vi "TestOutputToFileAPI.vi"() -> ()   [LabVIEW 2014, in "OutputToFileModule.lvlib"]
uses:
  OutputToFileModule.lvlib
  EventPlugins/EventPluginBaseClass/TypeDefs/clEvtReportArray.ctl
  EventPlugins/EventPluginBaseClass/TypeDefs/clEvtReport.ctl
  NetworkImpairmentModule/PublicAPI/Arguments/Broadcasts/dblNetworkTime.ctl
  NetworkImpairmentModule/PublicAPI/Arguments/Broadcasts/dblPktLoss.ctl
  OutputToFilePlugins/OutputToFileBasePlugin/Typedefs/PmuCfgOpt.ctl
  <userlib>/NIST/ModuleAdminLib/ModuleAdmin/ModuleAdmin.lvclass
  PublicAPI/Arguments/Broadcasts/clDidInit.ctl
  <userlib>/NIST/ModuleAdminLib/ModuleAdmin/ModuleAdmin.lvclass/ModuleAdmin.ctl
  PublicAPI/Arguments/Requests/clStopArgument.ctl
  PublicAPI/Arguments/Broadcasts/clStatUpdate.ctl
  PublicAPI/Arguments/Broadcasts/clErrorRpt.ctl
  <userlib>/NIST/ModuleAdminLib/ModuleAdmin/Accessors/Read CloneRegRef.vi
  <userlib>/NIST/ModuleAdminLib/CloneRegistration/CloneRegistration.lvclass
  OutputToFilePlugins/OutputToFileBasePlugin/OutputToFileBasePlugin.lvclass
  EventPlugins/EventPluginBaseClass/EventPluginBaseClass.lvclass
  NetworkImpairmentModule/NetworkImpairmentModule.lvlib
panel:
  in  "Show Panel":bool=TRUE
  in  "btnOutputErrorFile":bool
  in  "btnReadOutputPath":bool
  out "OutputPath":path
  in  "OutputPath":path
  in  "btnWriteOutputPath":bool
  in  "btnReadPmuConfig":bool
  out "clConfigOptions":T1={"TIME_BASE"=1000000, "STN"="Bus_1", "IDCODE"=0, "rdoPolRect"=enum."Rectangular", "rdoFloatInt"=enum."Float", "PHUNIT"=1000000, "rdoFreqDfreq"=enum."Float", "CHNAM"=[], "chkCfg2Prefix"=TRUE} caption="PMU Configuration Options" {"PHUNIT" max=16777216 step=1 format="%08d"; "IDCODE" format="%02x"; "TIME_BASE" max=16777216 step=1 format="%08d"}
  in  "btnWritePmuConfig":bool
  in  "clConfigOptions 2":T1={"TIME_BASE"=1000000, "STN"="Bus_1", "IDCODE"=0, "rdoPolRect"=enum."Rectangular", "rdoFloatInt"=enum."Float", "PHUNIT"=1000000, "rdoFreqDfreq"=enum."Float", "CHNAM"=["VA"], "chkCfg2Prefix"=TRUE} caption="PMU Configuration Options" {"PHUNIT" max=16777216 step=1 format="%08d"; "IDCODE" format="%02x"; "TIME_BASE" max=16777216 step=1 format="%08d"}
  in  "btnWritePktLoss":bool
  in  "btnWriteNetTime":bool
  in  "dblPktLoss":T2
  in  "dblNetworkTime":T3
  in  "btnWriteImpairRpt":bool
  in  "clPmuImpairRptArray":T4=[{"Timestamp"=1.0, "Synx"=[99.0+0.0i], "Freq"=59.0, "ROCOF"=0.0, "ID"=0}] {"Synx" format="%#_4g"}
  in  "btnWriteEvtRpt":bool
  in  "clEvtReportArray":T4=[{"Timestamp"=1.0, "Synx"=[100.0+0.0i], "Freq"=60.0, "ROCOF"=0.0, "ID"=0}] {"Synx" format="%#_4g"}
  in  "btnReadPlugin":bool
  out "PathToPluginIniFile":path=path "P:/Framework/PmuImpairment/PmuImpairPlugins/C37PmuImpairPlugin/C37PmuImpairPlugin.ini"
  in  "btnLoadPlugin":bool
  in  "PathToPluginIniFile":path=path "D:/Projects/PARTF/Framework/OutputToFile/OutputToFilePlugins/OutputToFileBasePlugin/OutputToFileBasePlugin.ini"
  in  "btnRemove":bool
  out "Status Log":string
  out "Active Modules (Array)":string[](array[string])
  in  "btnAdd":bool
  in  "btnStop":bool
  in  "Select Module":i32(ring)=-1 caption="Select Module to send Request" items=["All"=-1, "4140002"=4140002]
  # "Hidden"
  # "Visible"
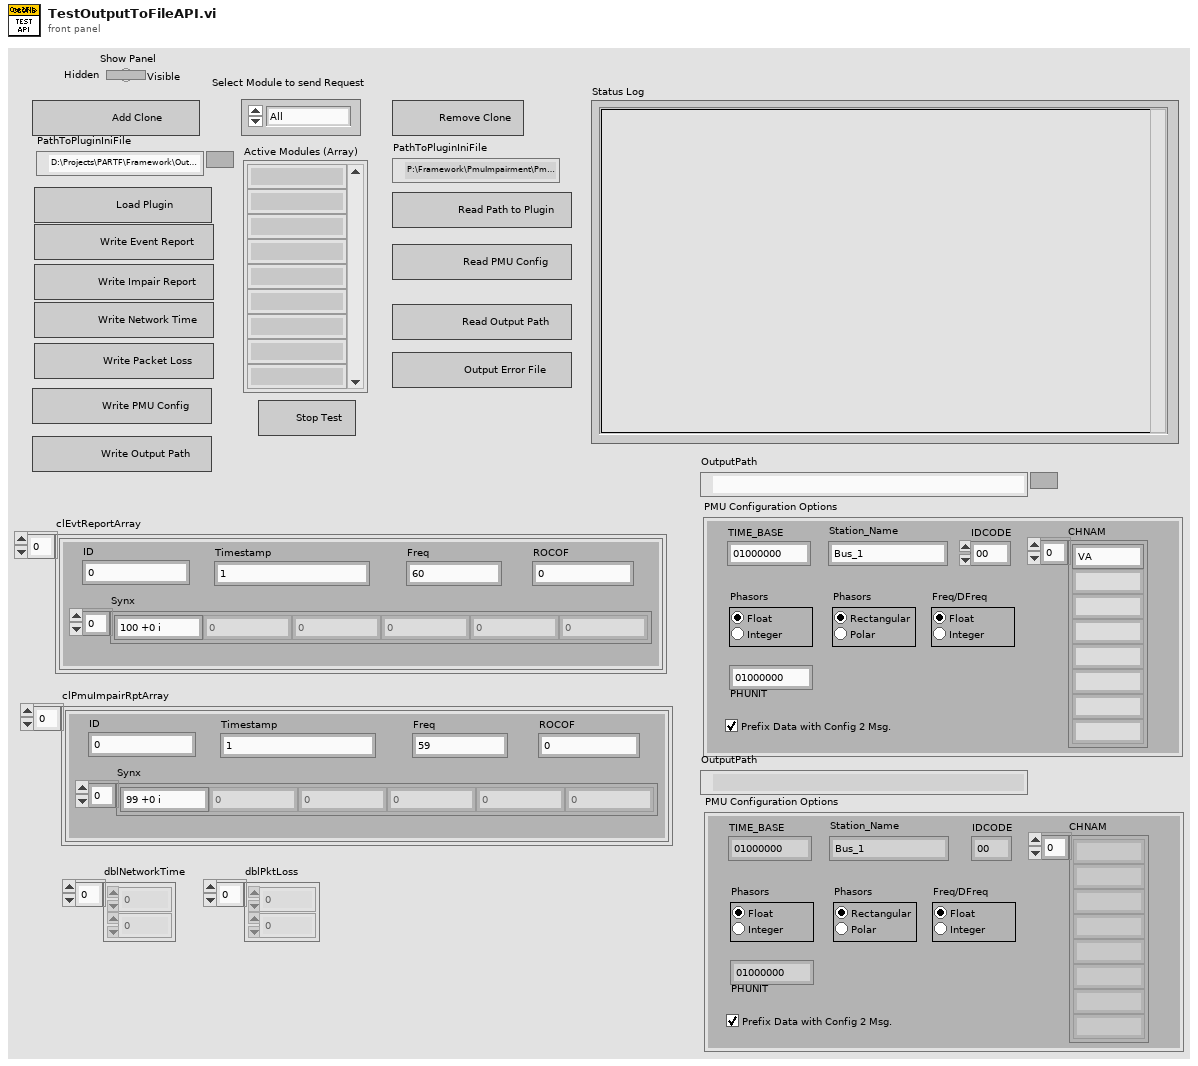
[diagram p1: front panel]
types:
  T1 = typedef "OutputToFilePlugins.lvlib/OutputToFileBasePlugin.lvclass/PmuCfgOpt.ctl" = cluster{"TIME_BASE":u64, "STN":string, "IDCODE":u16, "rdoPolRect":enum32{"Rectangular", "Polar"}, "rdoFloatInt":enum32{"Float", "Integer"}, "PHUNIT":u64, "rdoFreqDfreq":enum32{"Float", "Integer"}, "CHNAM":string[], "chkCfg2Prefix":bool}
  T2 = typedef "NetworkImpairmentModule.lvlib/dblPktLoss.ctl" = dbl[]
  T3 = typedef "NetworkImpairmentModule.lvlib/dblNetworkTime.ctl" = dbl[]
  T4 = typedef "EventPlugins.lvlib/EventPluginBaseClass.lvclass/clEvtReportArray.ctl" = T5[]
  T5 = typedef "EventPlugins.lvlib/EventPluginBaseClass.lvclass/clEvtReport.ctl" = cluster{"Timestamp":dbl, "Synx":cdb[], "Freq":dbl, "ROCOF":dbl, "ID":i16}
  T6 = typedef "OutputToFileModule.lvlib/clBroadcastEvents.ctl" = cluster{"DidInit":refnum<user-event>, "StatusUpdate":refnum<user-event>, "ErrorReport":refnum<user-event>, "DidStop":refnum<user-event>, "PathToPlugin":refnum<user-event>, "PmuConfig":refnum<user-event>, "OutputPath":refnum<user-event>}
  T7 = typedef "OutputToFileModule.lvlib/clDidInit.ctl" = cluster{"Init?":bool, "ModuleAdmin":refnum<class "ModuleAdmin.lvclass">}
  T8 = typedef "OutputToFileModule.lvlib/clStopArgument.ctl" = cluster{"Exit via Stop Module Req?":bool, "Wait for Module to stop?":bool, "ModuleAdmin":refnum<class "ModuleAdmin.lvclass">}
  T9 = typedef "OutputToFileModule.lvlib/clStatUpdate.ctl" = cluster{"Status":string}
  T10 = typedef "OutputToFileModule.lvlib/clErrorRpt.ctl" = cluster{"error":errorcluster, "AdditionalInfo":string}
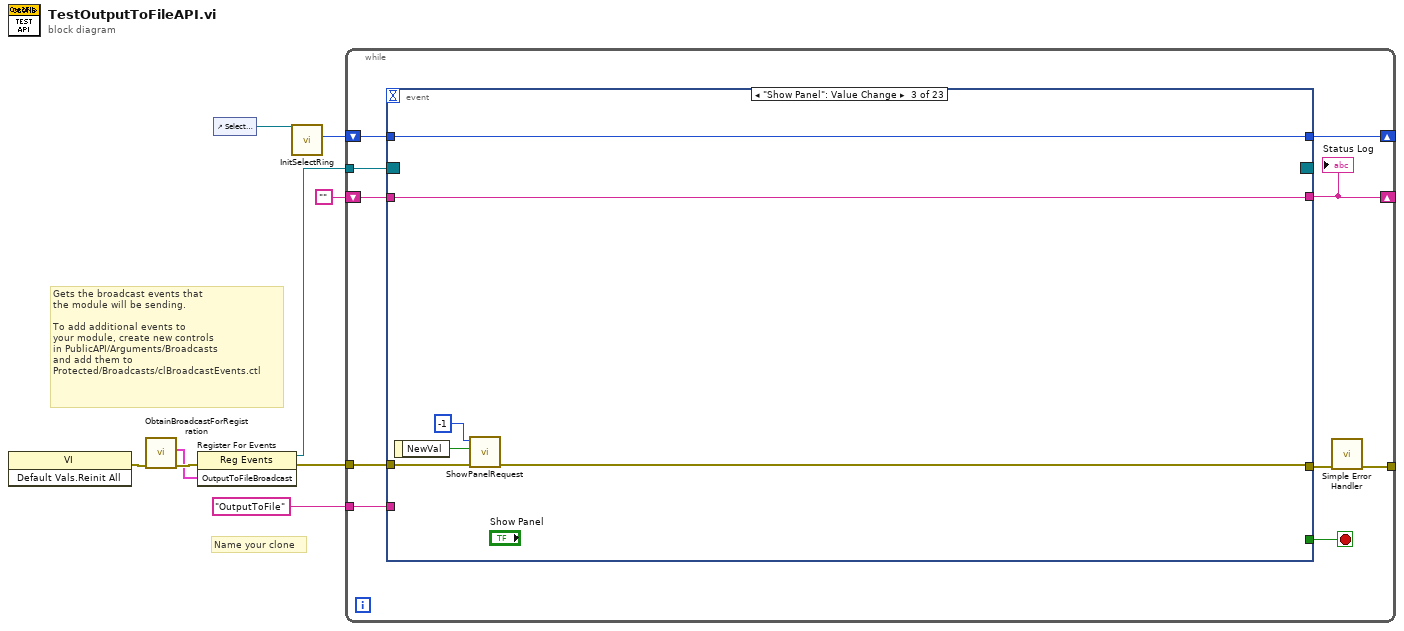
[diagram p0: block diagram]
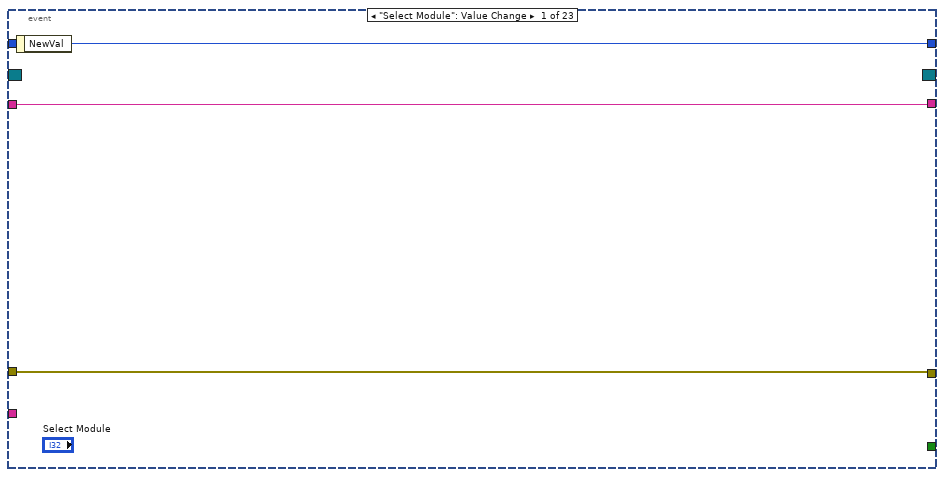
[diagram p2: hidden frame]
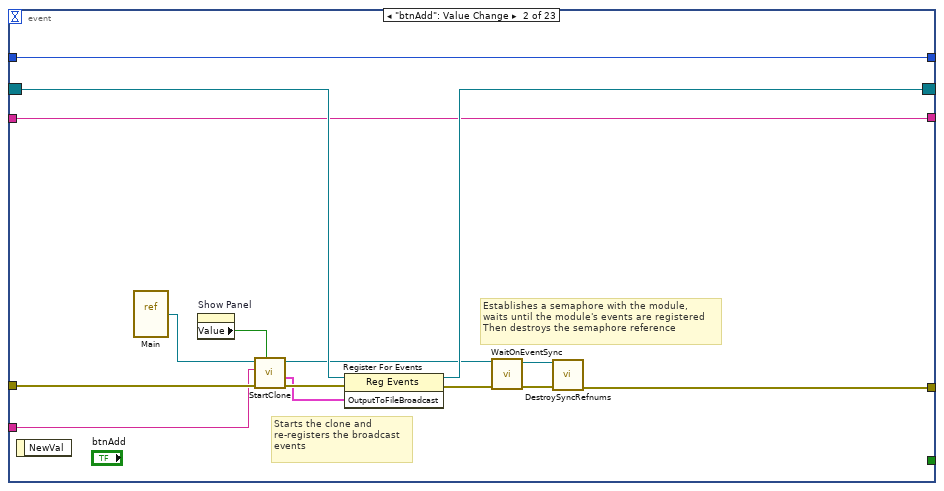
[diagram p3: hidden frame]
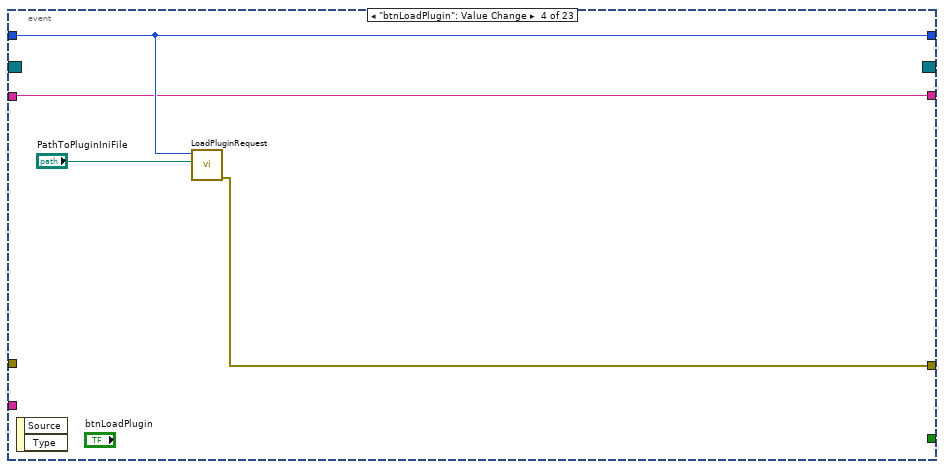
[diagram p4: hidden frame]
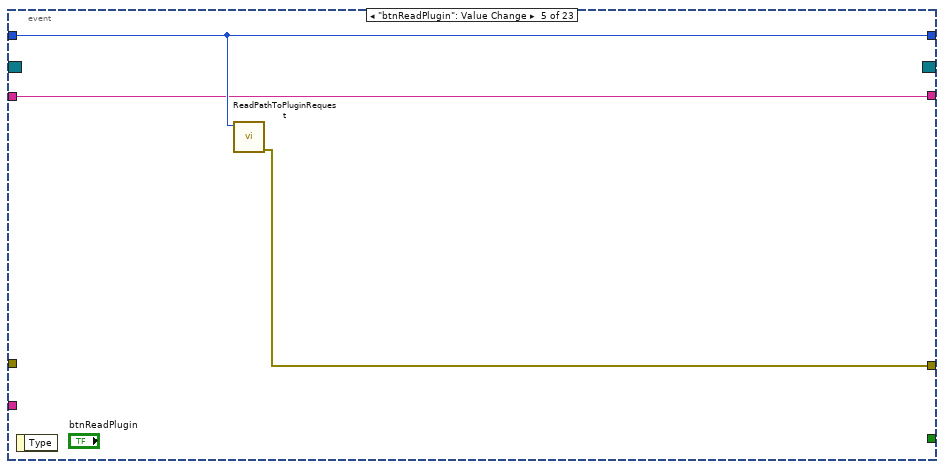
[diagram p5: hidden frame]
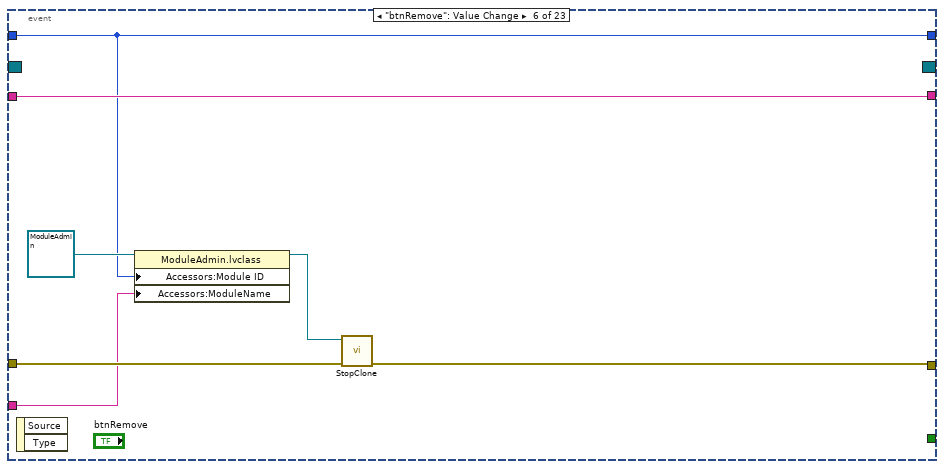
[diagram p6: hidden frame]
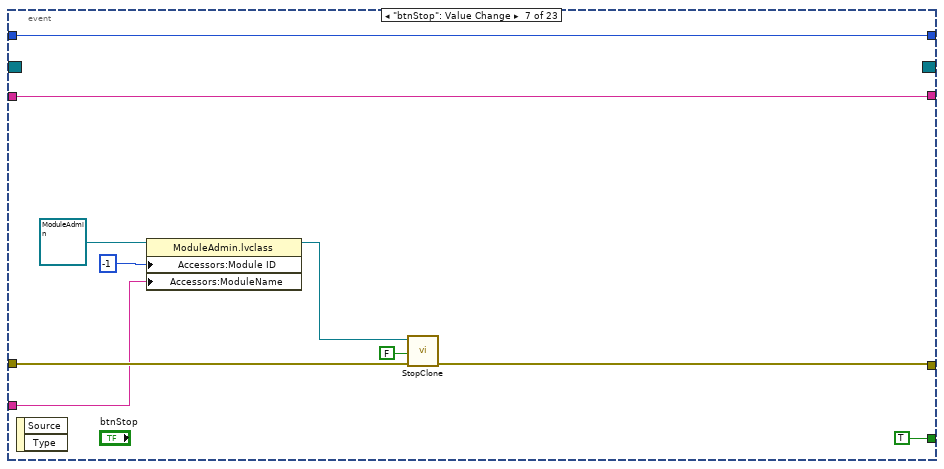
[diagram p7: hidden frame]
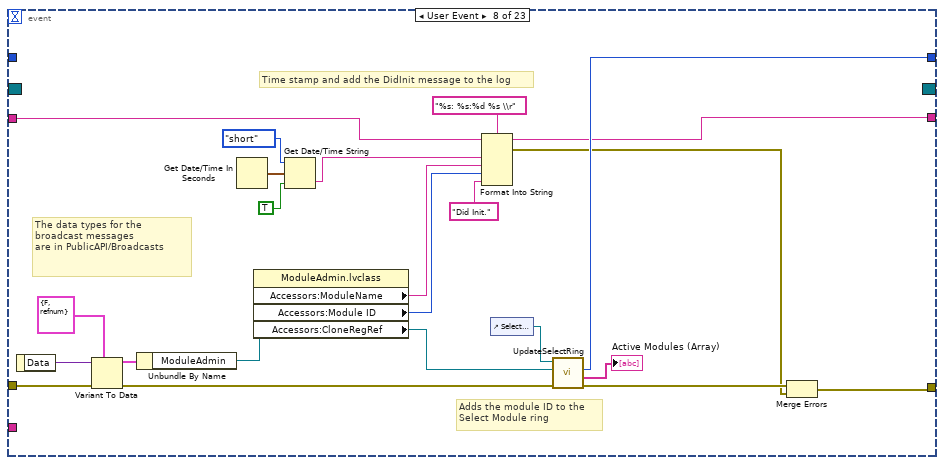
[diagram p8: hidden frame]
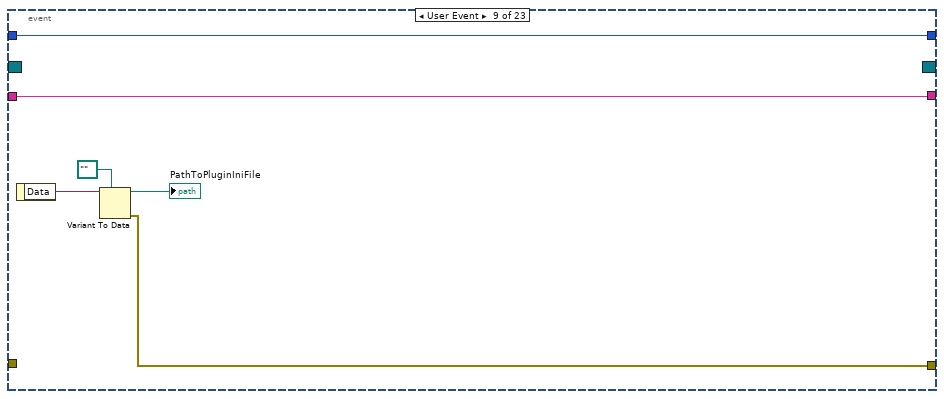
[diagram p9: hidden frame]
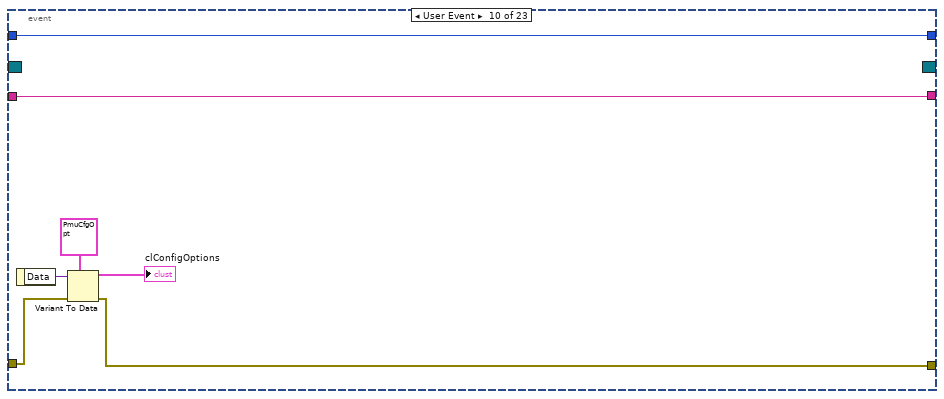
[diagram p10: hidden frame]
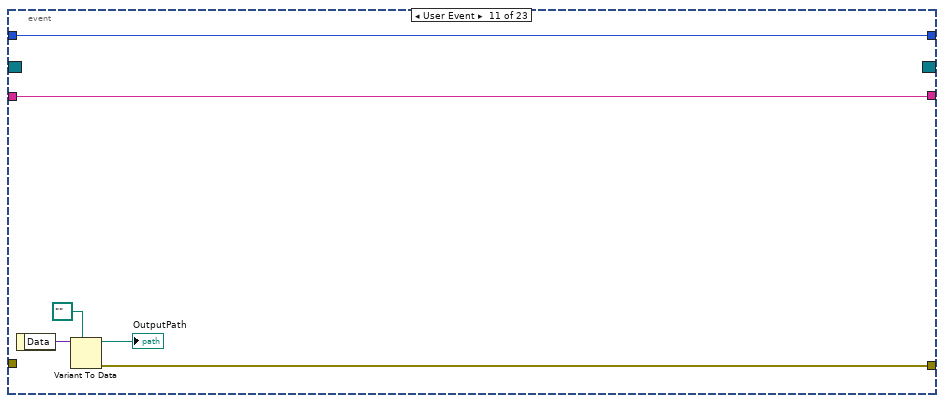
[diagram p11: hidden frame]
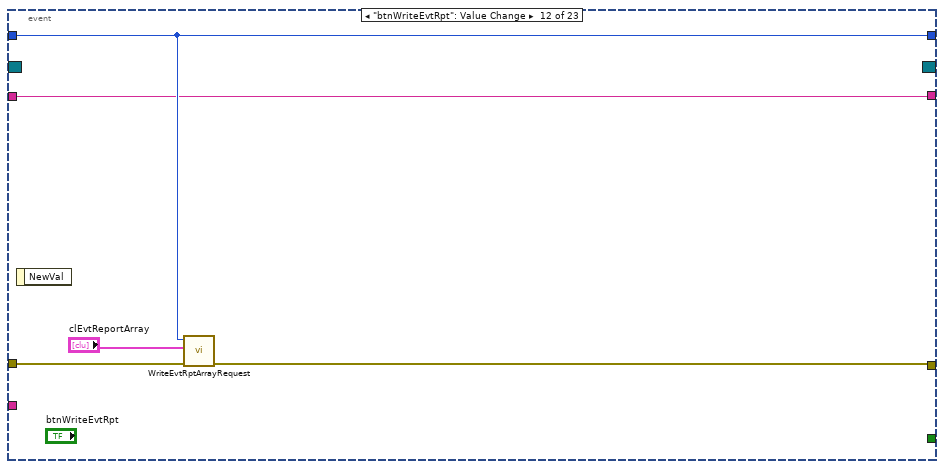
[diagram p12: hidden frame]
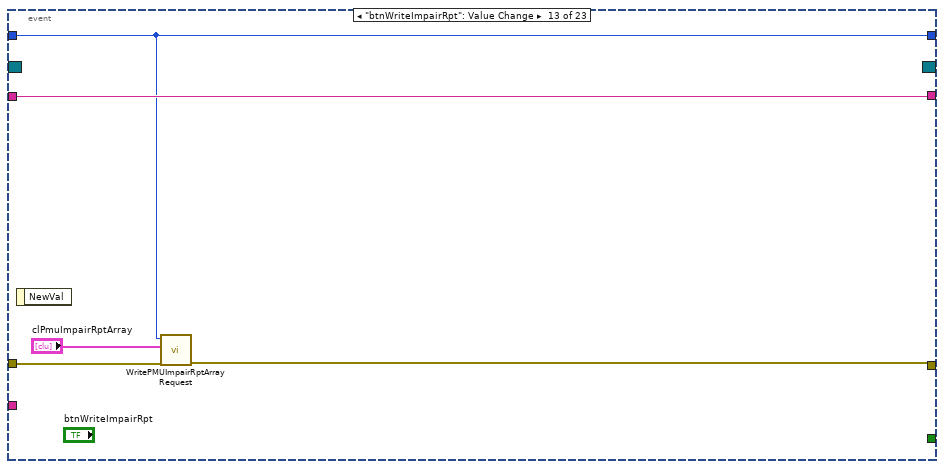
[diagram p13: hidden frame]
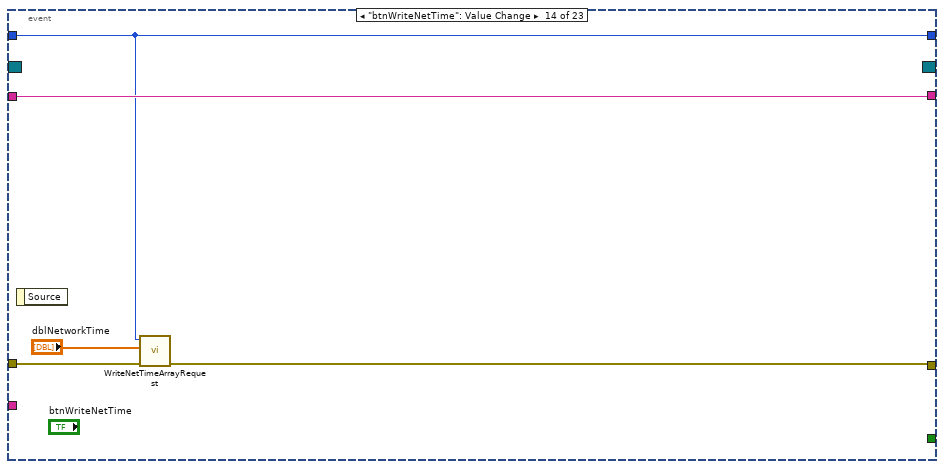
[diagram p14: hidden frame]
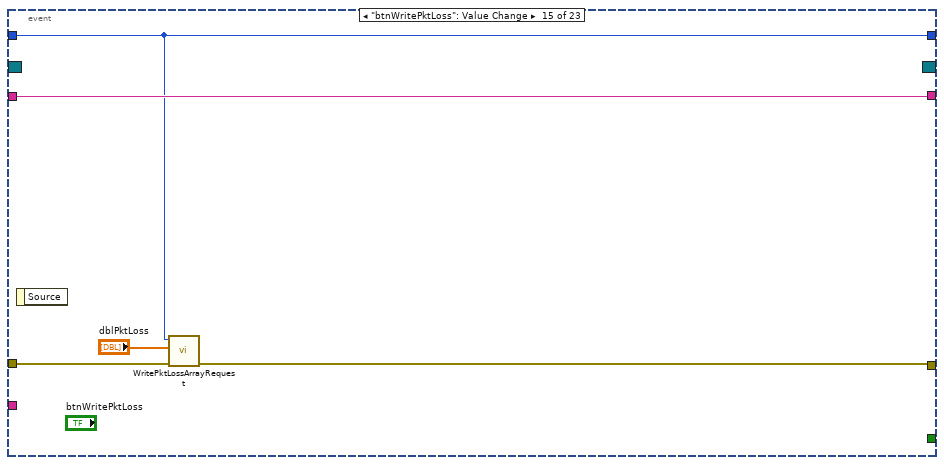
[diagram p15: hidden frame]
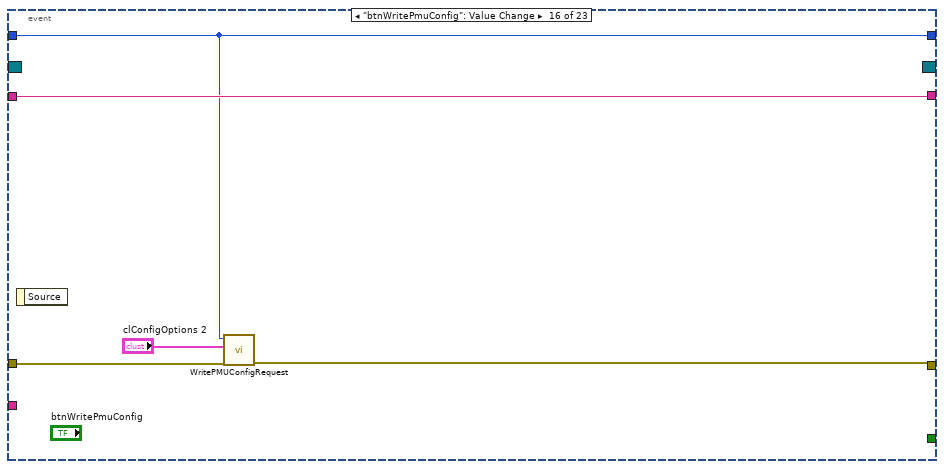
[diagram p16: hidden frame]
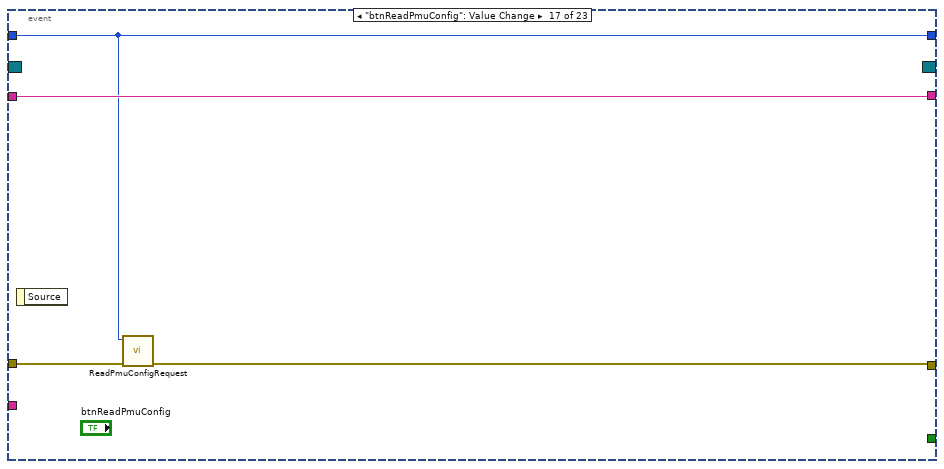
[diagram p17: hidden frame]
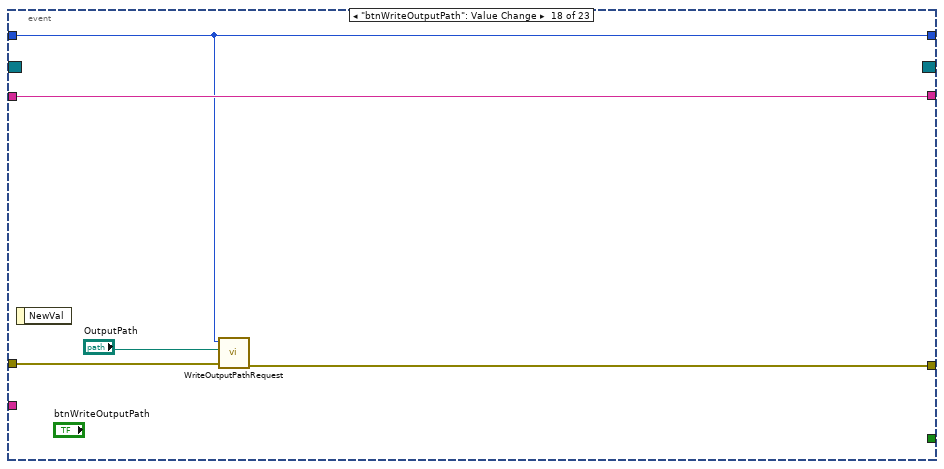
[diagram p18: hidden frame]
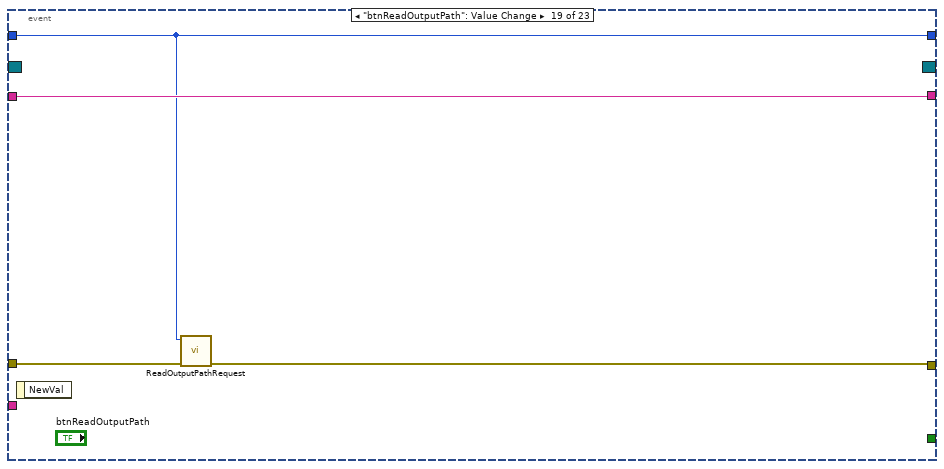
[diagram p19: hidden frame]
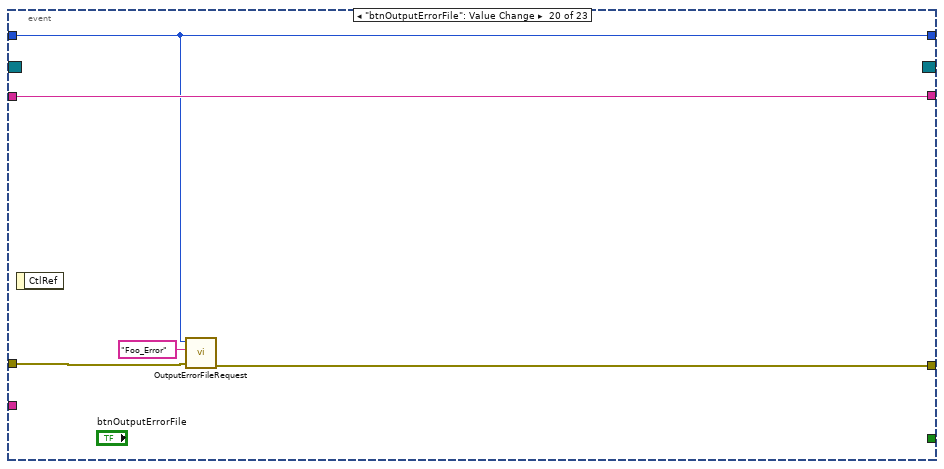
[diagram p20: hidden frame]
diagram:
  # "Name your clone"
  # "Gets the broadcast events that\nthe module will be sending.\n\nTo add additional events to\nyour module, create new controls\nin PublicAPI/Arguments/Broadcasts\nand add them to\nProtected/Broadcasts/clBroadcastEvents.ctl"
  n1 = invoke class="VI" method="Default Vals.Reinit All"() -> (error out=w7:errorcluster)  [unwired: 3 in, 2 out]
  n2 = call "ObtainBroadcastForRegistration.vi"("error in (no error)"=w7) -> ("error out"=w6:errorcluster, "OutputToFileBroadcast"=w5:T6)  [unwired: 9 in]
  n3 = register-events(error in=w6, w5) -> (reference out=w3:refnum<event-registration>, error out=w4:errorcluster)  [unwired: 1 in]
  n4 = control-ref of="Select Module"() -> (w9:refnum<vi>)
  n5 = call "InitSelectRing.vi"("Ring Refnum"=w9) -> ("Module Ring Value"=w8:i32)  [unwired: 9 in, 1 out]
  n6 = while {
    shift-right: [w18] -> _
    shift-left: w8 -> [w19]
    tunnel: w4 -> [w16]
    tunnel: w3 -> [w13]
    tunnel: [w14] -> _
    shift-right: [w12] -> _
    shift-left: "" -> [w11]
    tunnel: "OutputToFile" ("ModuleName") -> [w10]
    stop <- w17 stop-if-true
    n7 = event shown="[2] \"Show Panel\": Value Change" {
      selector: w13 -> [_ w29 _ _ _ _ _ _ _ _ _ _ _ _ _ _ _ _ _ _ _ _ _]
      dyn-events: [_ w28 _ _ _ _ _ _ _ _ _ _ _ _ _ _ _ _ _ _ _ _ _] -> _
      timeout: _ -> [_ _ _ _ _ _ _ _ _ _ _ _ _ _ _ _ _ _ _ _ _ _ _]
      tunnel: w19 -> [_ w37 w38 w46 w50 w53 w67 _ w96 w103 w108 w111 w115 w120 w126 w131 w135 w140 w145 w151 _ w193 w195]
      tunnel: [w22 w37 w38 w46 w50 w53 w67 w85 w96 w103 w108 w111 w115 w120 w126 w131 w135 w140 w145 w151 w162 w193 w195] -> w18
      tunnel: [_ _ _ _ _ _ TRUE _ _ _ _ _ _ _ _ _ _ _ _ _ _ _ _] -> w17
      tunnel: w16 -> [w20 w36 w43 _ _ w56 w65 w90 _ w97 _ w114 w118 w124 w128 w133 w138 w141 w146 w148 w171 w190 w202]
      tunnel: [w20 w30 w40 w44 w48 w55 w63 w74 w91 w98 w104 w113 w117 w123 w125 w130 w137 w139 w144 w149 w159 w182 w201] -> w15
      tunnel: [w21 w26 w39 w45 w49 w57 w62 w78 w95 w102 w107 w110 w119 w121 w129 w134 w136 w143 w147 w152 w168 w185 w194] -> w12
      tunnel: w11 -> [w21 w26 w39 w45 w49 w57 w62 w77 w95 w102 w107 w110 w119 w121 w129 w134 w136 w143 w147 w152 w169 w192 w194]
      tunnel: w10 -> [_ w25 _ _ _ w52 w59 _ _ _ _ _ _ _ _ _ _ _ _ _ _ w178 _]
      event "Select Module": Value Change {
        n8 = event-data() -> ("NewVal"=w22:i32)  [unwired: 1 in]
      }
      event "btnAdd": Value Change {
        # "Establishes a semaphore with the module,\nwaits until the module's events are registered\nThen destroys the semaphore reference"
        # "Starts the clone and\nre-registers the broadcast \nevents"
        n9 = event-data() -> ()  [unwired: 1 in, 1 out]
        n10 = vi-ref "Main.vi"() -> (w27:refnum<vi>)
        n11 = property on="Show Panel" class="Bool (strict)"() -> ("Value"=w23:bool)  [unwired: 2 in, 2 out]
        n12 = call "StartClone.vi"("ShowPanel?"=w23, "error in (no error)"=w36, "ModuleName"=w25, "VI Refnum"=w27) -> ("error out"=w35:errorcluster, "clBroadcastEvents"=w31:T6, "ModuleAdmin"=w24:refnum<class "ModuleAdmin.lvclass">)  [unwired: 5 in]
        n13 = register-events(reference=w29, error in=w35, w31) -> (reference out=w28:refnum<event-registration>, error out=w34:errorcluster)
        n14 = call <userlib>:"WaitOnEventSync.vi"("error in (no error)"=w34, "ModuleAdmin"=w24) -> ("error out"=w33:errorcluster, "ModuleAdmin"=w32:refnum<class "ModuleAdmin.lvclass">)  [unwired: 8 in]
        n15 = call <userlib>:"DestroySyncRefnums.vi"("error in (no error)"=w33, "ModuleAdmin"=w32) -> ("error out"=w30:errorcluster)  [unwired: 9 in]
      }
      event "Show Panel": Value Change {
        n16 = event-data() -> ("NewVal"=w42:bool)  [unwired: 1 in]
        n17 = call "ShowPanelRequest.vi"("error in (no error)"=w43, "ShowPanel"=w42, "Numeric"=-1) -> ("error out"=w40:errorcluster)  [unwired: 8 in]
      }
      event "btnLoadPlugin": Value Change {
        n18 = event-data() -> ()  [unwired: 1 in, 2 out]
        n19 = call "LoadPluginRequest.vi"("PathToPlugin"="PathToPluginIniFile", "Numeric"=w46) -> ("error out"=w44:errorcluster)  [unwired: 9 in]
      }
      event "btnReadPlugin": Value Change {
        n20 = event-data() -> ()  [unwired: 1 in, 1 out]
        n21 = call "ReadPathToPluginRequest.vi"("ModuleID"=w50) -> ("error out"=w48:errorcluster)  [unwired: 10 in]
      }
      event "btnRemove": Value Change {
        n22 = event-data() -> ()  [unwired: 1 in, 2 out]
        n23 = property class="ModuleAdmin.lvclass"(reference=refnum<class "ModuleAdmin.lvclass"> refnum ("NistModuleAdmin.lvlib:NistModuleAdmin.lvclass"), "Accessors:Module ID"=w53, "Accessors:ModuleName"=w52) -> (reference out=w51:refnum<class "ModuleAdmin.lvclass">)  [unwired: 1 in, 1 out]
        n24 = call "StopClone.vi"("error in (no error)"=w56, "ModuleAdmin"=w51) -> ("error out"=w55:errorcluster)  [unwired: 9 in]
      }
      event "btnStop": Value Change {
        n25 = event-data() -> ()  [unwired: 1 in, 2 out]
        n26 = property class="ModuleAdmin.lvclass"(reference=refnum<class "ModuleAdmin.lvclass"> refnum ("NistModuleAdmin.lvlib:NistModuleAdmin.lvclass"), "Accessors:Module ID"=-1 ("Module ID"), "Accessors:ModuleName"=w59) -> (reference out=w58:refnum<class "ModuleAdmin.lvclass">)  [unwired: 1 in, 1 out]
        n27 = call "StopClone.vi"("error in (no error)"=w65, "Wait for Module to stop?"=FALSE, "ModuleAdmin"=w58) -> ("error out"=w63:errorcluster)  [unwired: 8 in]
      }
      event User Event {
        # "Adds the module ID to the \nSelect Module ring"
        # "Time stamp and add the DidInit message to the log"
        # "The data types for the broadcast messages\nare in PublicAPI/Broadcasts"
        n28 = event-data() -> ("Data"=w89:variant)  [unwired: 1 in]
        n29 = Variant To Data(error in=w90, type=T7 {"Init?"=FALSE, "ModuleAdmin"=refnum} ("clDidInit"), Variant=w89) -> (data=w82:T7, error out=w87:errorcluster)
        n30 = Unbundle By Name(w82) -> ("ModuleAdmin"=w72:refnum<class "ModuleAdmin.lvclass">)
        n31 = Get Date/Time In Seconds() -> (seconds since 1Jan1904=w80:timestamp)
        n32 = property class="ModuleAdmin.lvclass"(reference=w72) -> ("Accessors:ModuleName"=w70:string, "Accessors:Module ID"=w69:i32, "Accessors:CloneRegRef"=w68:refnum<data-value>)  [unwired: 1 in, 2 out]
        n33 = Get Date/Time String(date format (0)=enum16{"short", "long", "abbreviated"}."short", seconds (now)=w80, want seconds? (F)=TRUE) -> (time string=w83:string)  [unwired: 1 out]
        n34 = Format Into String(format string="%s: %s:%d %s \\r", initial string=w77, w83, w70, w69, "Did Init.") -> (resulting string=w78:string, error out=w75:errorcluster)  [unwired: 1 in]
        n35 = control-ref of="Select Module"() -> (w86:refnum<vi>)
        n36 = call "UpdateSelectRing.vi"("error in (no error)"=w87, "CloneRegRef"=w68, "Ring Refnum"=w86) -> ("error out"=w76:errorcluster, "ActiveModules"=→"Active Modules (Array)":string[], "Module Ring Value"=w85:i32)  [unwired: 6 in]
        n37 = Merge Errors(w76, w75) -> (w74:errorcluster)
      }
      event User Event {
        n38 = event-data() -> ("Data"=w94:variant)  [unwired: 1 in]
        n39 = Variant To Data(type=path "", Variant=w94) -> (data=→"PathToPluginIniFile":path, error out=w91:errorcluster)  [unwired: 1 in]
      }
      event User Event {
        n40 = event-data() -> ("Data"=w101:variant)  [unwired: 1 in]
        n41 = Variant To Data(error in=w97, type=T1 {"TIME_BASE"=1000000, "STN"="Bus_1", "IDCODE"=0, "rdoPolRect"=enum."Rectangular", "rdoFloatInt"=enum."Float", "PHUNIT"=1000000, "rdoFreqDfreq"=enum."Float", "CHNAM"=[], "chkCfg2Prefix"=TRUE} ("clConfigOptions"), Variant=w101) -> (data=→"clConfigOptions":T1, error out=w98:errorcluster)
      }
      event User Event {
        n42 = event-data() -> ("Data"=w109:variant)  [unwired: 1 in]
        n43 = Variant To Data(type=path "", Variant=w109) -> (data=→"OutputPath":path, error out=w104:errorcluster)  [unwired: 1 in]
      }
      event "btnWriteEvtRpt": Value Change {
        n44 = event-data() -> ()  [unwired: 1 in, 1 out]
        n45 = call "WriteEvtRptArrayRequest.vi"("error in (no error)"=w114, "EvtRptArray"="clEvtReportArray", "ModuleID"=w111) -> ("error out"=w113:errorcluster)  [unwired: 8 in]
      }
      event "btnWriteImpairRpt": Value Change {
        n46 = event-data() -> ()  [unwired: 1 in, 1 out]
        n47 = call "WritePMUImpairRptArrayRequest.vi"("error in (no error)"=w118, "PmuImpairRptArray"="clPmuImpairRptArray", "ModuleID"=w115) -> ("error out"=w117:errorcluster)  [unwired: 8 in]
      }
      event "btnWriteNetTime": Value Change {
        n48 = event-data() -> ()  [unwired: 1 in, 1 out]
        n49 = call "WriteNetTimeArrayRequest.vi"("error in (no error)"=w124, "NetTimeArray"="dblNetworkTime", "ModuleID"=w120) -> ("error out"=w123:errorcluster)  [unwired: 8 in]
      }
      event "btnWritePktLoss": Value Change {
        n50 = event-data() -> ()  [unwired: 1 in, 1 out]
        n51 = call "WritePktLossArrayRequest.vi"("error in (no error)"=w128, "PktLossArray"="dblPktLoss", "ModuleID"=w126) -> ("error out"=w125:errorcluster)  [unwired: 8 in]
      }
      event "btnWritePmuConfig": Value Change {
        n52 = event-data() -> ()  [unwired: 1 in, 1 out]
        n53 = call "WritePMUConfigRequest.vi"("error in (no error)"=w133, "PmuConfig"="clConfigOptions 2", "ModuleID"=w131) -> ("error out"=w130:errorcluster)  [unwired: 8 in]
      }
      event "btnReadPmuConfig": Value Change {
        n54 = event-data() -> ()  [unwired: 1 in, 1 out]
        n55 = call "ReadPmuConfigRequest.vi"("error in (no error)"=w138, "ModuleID"=w135) -> ("error out"=w137:errorcluster)  [unwired: 9 in]
      }
      event "btnWriteOutputPath": Value Change {
        n56 = event-data() -> ()  [unwired: 1 in, 1 out]
        n57 = call "WriteOutputPathRequest.vi"("error in (no error)"=w141, "OutPath"="OutputPath", "ModuleID"=w140) -> ("error out"=w139:errorcluster)  [unwired: 8 in]
      }
      event "btnReadOutputPath": Value Change {
        n58 = event-data() -> ()  [unwired: 1 in, 1 out]
        n59 = call "ReadOutputPathRequest.vi"("error in (no error)"=w146, "ModuleID"=w145) -> ("error out"=w144:errorcluster)  [unwired: 9 in]
      }
      event "btnOutputErrorFile": Value Change {
        n60 = event-data() -> ()  [unwired: 1 in, 1 out]
        n61 = call "OutputErrorFileRequest.vi"("error in (no error)"=w148, "Filename"="Foo_Error", "ModuleID"=w151) -> ("error out"=w149:errorcluster)  [unwired: 8 in]
      }
      event User Event {
        # "Time stamp and add the Stop message to the log"
        # "The Stop Argument  is found in\nPublicAPI/Arguments/Requests"
        n62 = event-data() -> ("Data"=w170:variant)  [unwired: 1 in]
        n63 = Variant To Data(error in=w171, type=T8 {"Exit via Stop Module Req?"=FALSE, "Wait for Module to stop?"=FALSE, "ModuleAdmin"=refnum} ("Stop Argument"), Variant=w170) -> (data=w166:T8, error out=w165:errorcluster)
        n64 = Unbundle By Name(w166) -> ("ModuleAdmin"=w157:refnum<class "ModuleAdmin.lvclass">)
        n65 = property class="ModuleAdmin.lvclass"(reference=w157) -> ("Accessors:ModuleName"=w155:string, "Accessors:Module ID"=w154:i32, "Accessors:CloneRegRef"=w153:refnum<data-value>)  [unwired: 1 in, 2 out]
        n66 = Get Date/Time In Seconds() -> (seconds since 1Jan1904=w173:timestamp)
        n67 = Get Date/Time String(date format (0)=enum16{"short", "long", "abbreviated"}."short", seconds (now)=w173, want seconds? (F)=TRUE) -> (time string=w175:string)  [unwired: 1 out]
        n68 = Format Into String(format string="%s: %s:%d %s \\r", initial string=w169, w175, w155, w154, "Stopping") -> (resulting string=w168:string, error out=w160:errorcluster)  [unwired: 1 in]
        n69 = control-ref of="Select Module"() -> (w164:refnum<vi>)
        n70 = call "UpdateSelectRing.vi"("error in (no error)"=w165, "CloneRegRef"=w153, "Ring Refnum"=w164) -> ("error out"=w161:errorcluster, "ActiveModules"=w163:string[], "Module Ring Value"=w162:i32)  [unwired: 6 in]
        n71 = local write "Active Modules (Array)"(w163) -> ()
        n72 = Merge Errors(w161, w160) -> (w159:errorcluster)
      }
      event User Event {
        # "Time stamp and add the Status message to the log"
        # "The data types for the broadcast messages\nare in PublicAPI/Broadcasts"
        n73 = event-data() -> ("ModuleID"=w177:i32, "Data"=w189:variant)  [unwired: 1 in]
        n74 = Variant To Data(error in=w190, type=T9 {"Status"=""} ("clStatUpdate"), Variant=w189) -> (data=w187:T9, error out=w184:errorcluster)
        n75 = Get Date/Time In Seconds() -> (seconds since 1Jan1904=w186:timestamp)
        n76 = Unbundle By Name(w187) -> ("Status"=w176:string)
        n77 = Get Date/Time String(date format (0)=enum16{"short", "long", "abbreviated"}."short", seconds (now)=w186, want seconds? (F)=TRUE) -> (time string=w179:string)  [unwired: 1 out]
        n78 = Format Into String(format string="%s: %s:%d %s \\r", initial string=w192, w179, w178, w177, w176) -> (resulting string=w185:string, error out=w183:errorcluster)  [unwired: 1 in]
        n79 = Merge Errors(w184, w183) -> (w182:errorcluster)
      }
      event User Event {
        # "#CodeNeeded\nThis is a very crude error handler\nA better error handler will be needed"
        # "The data types for the broadcast messages\nare in PublicAPI/Broadcasts"
        n80 = event-data() -> ("ModuleID"=w198:i32, "Data"=w203:variant)  [unwired: 1 in]
        n81 = Variant To Data(error in=w202, type=T10 {"error"={"status"=FALSE, "code"=0, "source"=""}, "AdditionalInfo"=""} ("Cluster"), Variant=w203) -> (data=w199:T10, error out=w201:errorcluster)
        n82 = Unbundle By Name(w199) -> ("error"=w197:errorcluster)
        n83 = Number To Decimal String(number=w198) -> (decimal integer string=w196:string)  [unwired: 1 in]
        n84 = call <vilib>:"General Error Handler.vi"("[error source] (\" \")"=w196, "error in (no error)"=w197) -> ()  [unwired: 9 in, 5 out]
      }
    }
    "Status Log" <- w12
    n85 = call <vilib>:"Simple Error Handler.vi"("error in (no error)"=w15) -> ("error out"=w14:errorcluster)  [unwired: 4 in, 4 out]
  }
